vi "Main_21b.vi"() -> ()   [LabVIEW 2023]
uses:
  Cluster_Node.ctl
  ENUM Tile Marks.ctl
panel:
  out "left of set":i32
  out "Left of count":i32
  out "Array":T1[][](array[typedef])
  out "Start Point":T2
  out "Answer":i32
  in  "Puzzle":string="...................................................................................................................................\n.....#..#..#.#..#..#..#................##.#.......#....................#......#.##...........#.....##...................#........#.\n.....#.#.............#.............#.....#.........#..................................#......#....#...##...#.#........#......###...\n.......#...#................#.......#....#.....#...#.......................#......#...#.##...#.....#.........#.......#.#...........\n.##.............#...................#...#......#........#.........................#...#........#....#....#.........#..........#....\n.....#..##....#..#...#......##......#.................................................#.#.....#......#......#.#.##.................\n..............#......#......#................#.................#.................#................#..#...#........##.............#.\n..........##..........##.......#.#.....#..........#...#.........#.....................#....#....................#..#.....##..#..##.\n.#.#..#..#.#....#....#.....#...#.#.................................................#......................#..##..#.........#...#...\n.....................#.........#.......###..#......................#...........####........##.......#.#.#......#.#....##.....#...#.\n.#.#...#....#.........##...#...........#..##.......#.......#.......#................#.....#...#...#.#.....#..............##......#.\n................#...#..#.........#.##............................................#......##.....##.......#...#........#..#..#.......\n..#..#..####...###.#..........#........#.......#.............#.....#....#............#..#........##......##.......#.....#....#.....\n.......#..........#.......................#.............##..........#..#..........#.....#.............##.........#..............#..\n..................#.............##...........................#.#......##.......................##.....#.#.....#................#...\n.......#...................##........#...............................#..............#..#..#.#..#..........#........#...........#...\n...#..........#..#...#.#.#............................#......................#.......#......##...#...............#...#..#..........\n...#.#..........#.#.....#........#.....#...#.......................#.....#..#...............#.....#.#......#....##...#....#..###...\n...#.##........#..##...#..........#..#..................................#..#.#.#.........#...........#....#.....#...#.#.........#..\n.....#.......#........#..............#.##.............#..#........#....#.....#.............#....#.#.#........##........#...#..#....\n....#......##....##........#..#....##.................#......................#.#.#................#....#..###..#...#...............\n....#....#.#........#.......#........#...................#.....#.........#....#............##.........#..............#...........#.\n............#..#.##..................#..........##.........................#..#....#................#................#..#....#.....\n.##.##........#..###.......#....#......................##..#......#.....#...#..#...............##.#.....##........#................\n.......#..#........#.........#...................#..#.....##...............#.#.#...#..........#............#.....##.........#......\n...###.......#...............#...................#..#...##.........#.............##..#..........................#..#...#.....#.....\n..#..............##.........#..#...............................#........#......#.#....#..........#................##.#...#.........\n...#......#..#....#.........#..#..........##............#....#.........#....#..#......#.........#..#...........#...................\n.#...###.....................#.............#.......#......###..#...........#.........................#..#.......#.#..#.....#.......\n.###........#......##...#...........................##......#.........#.........#........#........#.....##..........#....#.........\n.......#........#..#......#..............#..........##...#...#...........................#...........#...#..#......#...........#...\n.#....#........#......#..##..................#....................#.................................#......#.....#..#.......#......\n...#........#.....#..##...#.#.............#...#.#.#.....#......#........#...........#....#...............#..#.....#.......#........\n....#....#...#.#....#................#..#......#........#.#........#..#.#..#..#.....#..#..................##...................#...\n.......##........#...#..............###.#....#....#..#....##...#....##.#............#..#.#...#............#...................#.#..\n..#......#.........#..#.................#...#.......#....#...#..............##...#..........#.#...........................#....#...\n..#......#..#...........................#...........#....#.............#.#.........#...#.........................##............#...\n.....#................#.........#.#.........#...........#.#............#..................#....#.........................#..#..#...\n......#...#....##...................#.................#..#........#..#..#.....................#.............#.......#..#......#....\n.............##.................#.......#.........#..#....#...#.......#...................#.........#.......##.#...................\n......#....#.................#..#....#..##..#............#..............#.............#.....#..#..#................#..#...#......#.\n..................#.........#.....................#......#....##..##...##..........#......#......#..#.............#.....#....#.....\n.......#...#..#....#..........#.......#.#.#...##.....##.#....#.##..................##........#...##..................#.............\n.............#...#..................#......##.........#.......##......#...#....##.....#...#..#...................#...####..........\n.............................#.......#....#........#..........#...#.......#.#............#..###........#...........#.#.............\n..........#...................#..#...............#.#..................#.....#...#..............................................##..\n.........................................#...#.#....#.......#........#..#......#.........#...............#.........................\n......#...#.......................#.....#................#.........#..#......#....................####.#..#.....................##.\n.......#...................#.##....#......#..........#...............##...#...#...............#.......#.....#.................#....\n....#.#...##............#.......#..........#..................#..........#.........#........#.........##...#.......................\n...#......#.........#........#....#.....#.........#....##....#..................#.......#.#.........#.#..................##....#...\n.....#................#.#...........#.............#..#.......#..........#..#...#.#.....###......##.....#.#.#.#.................#...\n.....................#..##.##...#...............#..#....#....#....#..####...#..................................#.........##..#.....\n.......##...............#......#.....#..........#..#..#.#.............#.....#......#.#.......#..................#............#..##.\n...#............#...#.........##............#...#...#......#.......#.....#...##...##...#...#................................#......\n...#.#.............................................##..............##..................#...........#...#..........#...........##...\n...#.#....................#......#....#.....##..........#.........#......#.#.......##.#.#....#.#....#.....#....##..................\n.............#...#.#..#......#........#.#...##.#...............#....#.........................#....#.......#.....##...#.........#..\n..................##..#..###......................#.......#.##.....#....#..#.....#....#..............#.....#.#..#....#.............\n.............#......#.###..###........#.#.#......#.#....#..#.......#..#............#.........#.#..#...............#.............##.\n.............#...#.............#.#.#..##..####..#......#.##.#...........##...##.............#......#.............#..#............#.\n..........#........#......#.#........#..............#......#..#.#.....#.................#...#...............#.#..........##........\n..............#.............##.....#............................#..........#..........#..#.....................#..#..#.............\n..........#...#.#.......##....#.......#..##......#...#.....#............#................#....#.......................#............\n....................#.....#..........#.......#.#........#...##..............#.....#.......#..##...#..#####.#.#.........##....#.....\n.................................................................S.................................................................\n........#.........##....#........#...........................##........#..............#........#.....#.#..............#....#.......\n......#............#.............#............#.##...........#..#.....#....#.....#......#.#.#.......#.#.#...#......................\n............................#.........#........###........#...#....#.........#................#..#.............#....#..............\n............#......##..##.##...##.............#.........#............#.###.....#..................##..................#..#.........\n..............#......#................#...............#.....##..#..........#.....#..#..........#...........#.......................\n.........................#...........#..#......#.............#..#....#.......#..#.....#...#.............................#........#.\n...........##.....##.................#..........#.#.#..............#.....#.........#............#.................#................\n.........................#......#.....#...#.##...........#......#....#....#......#..#.#..#..###..##.##.....#...................#...\n.....#...........#.....#.......#..##......##.#.#.#..........#..#..............#...#.#.#.....#............#.#....#..............#.#.\n...#...........#.........#..#.#.#.........#........#..#........................#..........#.............#....##.#...............#..\n...............#.....................................#..............................##...###.................#..#..........#.....#.\n........#..........#..#......###............#........................#..........#............................................#.....\n...............................#....................#..................................##.............#............................\n.........#............#..#..........#........#..#...##....#....#..#......#.....#.#...#......................##..................#..\n......##.#..........##.#..................................#.........#......##..#...............#........#.....#............#.......\n.........#..................#...........#.#.......................#..........#.......##.......#.....#...##...#........#...#.#......\n...#...................#.....#...........##............#..#...#..................#.#..........#........................#...........\n..#.........#.........#.........##...#.....#...........#.....................#....#............#..#.......#.........#.....#........\n..........#....#..........#.........#..........#..###........#.#..........##.................#......#...#..............#...........\n..#....##..........................#..........#........#.#..##..#.....#.#....#..#.....................#............#.#...........#.\n.....................................#..#.#..#...........#...#.#.......#........#...#.........#...#..#...............#.............\n.........#.#....##.................#.#.....#....#..#..#................#...##.......#...........#.....#.................##.........\n..#.........................#......#..............#.............#.......#.............#........#................#...###.#........#.\n.#..#............#..............#..#...........#................#.........#....#................#..#.............#.....#...#.....#.\n.....#.......................#............#...............#..........###.....##...........#..#...#.##.........#.......#............\n.#..#..........#.............................#......#.......##..........#.........#....#...#.....#..........#....#.................\n.........#.......................#.##.....#.....#.#....#.......##.....#....#......#.......#.#.....................#.##..#..#....#..\n.#......#.....#.....#.....................##.........#....#...##..#..................##...#.#.#..#........#..#.........#.#....#.##.\n.#...............................#.#.#..#..##.....#........#...#.....#..#...#......#.#....#...##..................#................\n...........#......#...............#.....#.....#..##.........##........#.....#.........#...#..#............#.#.#...........#........\n..#............#..##..#..#..........#...#.......#.........#.......#.....#............................................#....#...#.#..\n....#...........#....................#............................#.#...#...............#.#..#.....................................\n.....##......#.##...#............................#........#...#...........#.........#......##...........#.#..#...............#.....\n......#..............##.#.###...........#.....#.#.##....#..#..........#...#..#..............................#.....#..............#.\n..##.....................##...............#...#......#........#..................#............................#.###..#...#....#..#.\n........#.#............#....................##.....#..........#...................#...#..#...........#........#.........#....##....\n.....#....#..#...............#............#.....#.......#...#........#............#..##.............#.......................#......\n..#.........#.............#...........................#.......#.#.................#..###.........................#.#.#.#.....#.....\n....#...#.................#................#........#..........#..........#.......#..........................#.#......#.......#....\n......#..##........#....#........................#.........#.........#................#......................#........#.....#....#.\n............#......#.........................................##......#.#..#.........#.............##..........#............#.......\n......#.#....#....#......#......##................#........#......#....#.....#....#.#..............#.......#.#...#......#......#...\n.....#............##.....#........#.#..#.........#.#................#...#.........#...........#.....#..#............#.....#..#.#...\n.......##..#........#..#..#.......................#............................................................#...#.#.....#.......\n....#...............#.......#............#.................#..............#..#...........#.......#............#................#...\n.......#.........##.......................#.......#....#......###...#....#..#................##...#.................#.#............\n...#.#.......#........#..#...........................#......#.....#.........##..........#..........##..............#....#........#.\n..#.#...........##..........#...#.........#..........#.#............##..................................#...........##.............\n.#..............#.........##.#.##..#...#....#.............#..............#............#..................#.#........#..............\n..#..#.....#....#.........#..#.#......#..#...#.............#..........#.................#...##.....#..........#...............#....\n......#.........#..#.#.....#................#......................#...##...........#..#................#.............#....##....#.\n...................#.....#.........##.....##...........................#....................#......#..................#..#.#.......\n..#............#...........##.#................................#............................#.........................#...#....#...\n.....#............#..............#......#..#....................#............................#....#....................#....#..#...\n..........#..#.#.#..............#.................................................................#...............##...........#...\n........##.................#..........#.....##....#.........#..#...#.##.....................#..#.........................#.......#.\n....##.........#.....#.....................#..#.##...........#..#.........................#..........#.....#........#....##......#.\n..............#.......#........#.......#..##...................#...#....................#...........#....#.........................\n...............#.............##......#.##.#............#...................#....#..............#...#..#.#.....#...............#....\n.....#..............#...#.......##..........#......#...#..................#..................#........#....#.........#.............\n.#.......#.#......#........................#..#......#......................#......##....##..#..........#...................#......\n..........#...........#..#..###........#.#......#.....................................#####.......##........#.....#.......#........\n..##................#............#..........#...##....#........................#....#........#....#.##......#.........##....#......\n.........#....#.....#....#.#...##..........#.........#.#.................##..............#..#......#.......#...#..............#.#..\n..................................................................................................................................."
  in  "Example":string="...........\n.....###.#.\n.###.##..#.\n..#.#...#..\n....#.#....\n.##..S####.\n.##..#...#.\n.......##..\n.##.#.####.\n.##..##.##.\n..........."
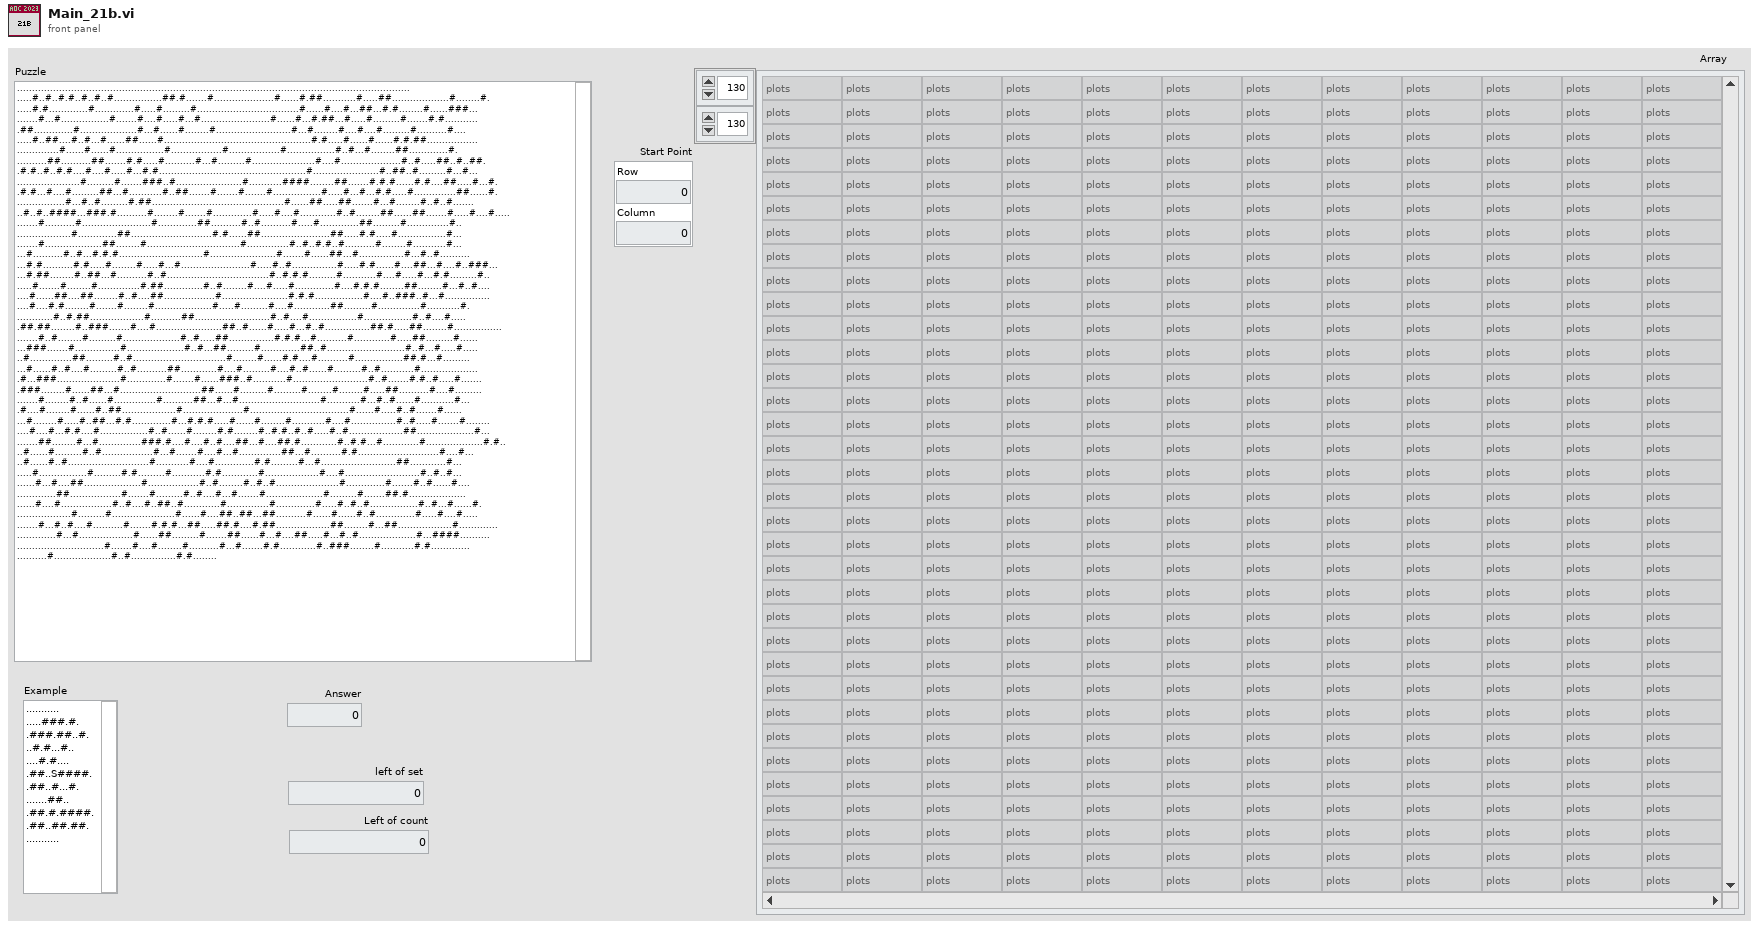
[diagram p1: front panel]
types:
  T1 = typedef "ENUM Tile Marks.ctl" = enum16{"plots", "rocks", "Start", "Marked Tiles"}
  T2 = typedef "Cluster_Node.ctl" = cluster{"Row":i32, "Column":i32}
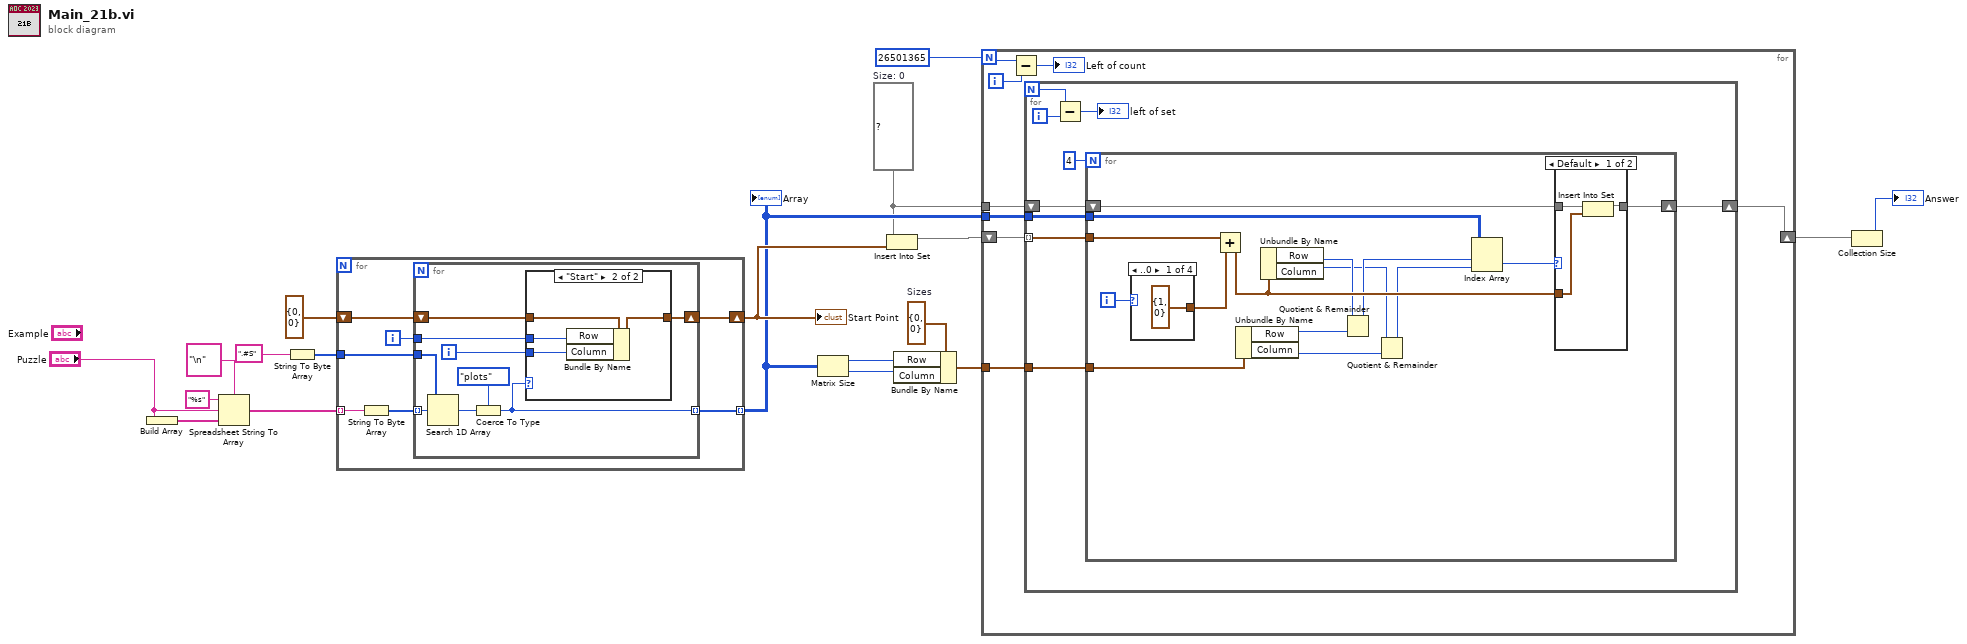
[diagram p0: block diagram]
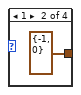
[diagram p2: hidden frame]
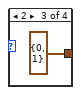
[diagram p3: hidden frame]
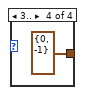
[diagram p4: hidden frame]
diagram:
  w8 = T2 {"Row"=0, "Column"=0}  # Sizes
  w7 = set{T2} {}  # Size: 0
  n1 = Build Array("Puzzle") -> (w19:string[])
  n2 = Spreadsheet String To Array(delimiter (Tab)="\n", format string="%s", spreadsheet string="Puzzle", array type (2D Dbl)=w19) -> (array=w16:string[])
  n3 = String To Byte Array(string=".#S" ("format string")) -> (unsigned byte array=w14:u8[])
  n4 = for {
    tunnel: w16 -> [w26] mode=indexing
    tunnel: w14 -> [w25]
    tunnel: [w23] -> w9 mode=indexing
    shift-right: [w20] -> w10
    shift-left: T2 {"Row"=0, "Column"=0} ("Point") -> [w22]
    i -> [w21]
    n5 = String To Byte Array(string=w26) -> (unsigned byte array=w24:u8[])
    n6 = for {
      tunnel: w25 -> [w35]
      tunnel: w24 -> [w34] mode=indexing
      tunnel: [w31] -> w23 mode=indexing
      shift-right: [w27] -> w20
      shift-left: w22 -> [w30]
      tunnel: w21 -> [w29]
      i -> [w28]
      n7 = Search 1D Array(1D array=w35, element=w34) -> (index of element=w33:i32)  [unwired: 1 in]
      n8 = Coerce To Type(0:w33, 1:ENUM_Tile_Marks."plots") -> (2:w31:T1)
      n9 = case shown="\"Start\"" w31 {
        tunnel: w30 -> [w36 w40]
        tunnel: w29 -> [_ w38]
        tunnel: w28 -> [_ w37]
        tunnel: [w36 w39] -> w27
        frame Default {
        }
        frame "Start" {
          n10 = Bundle By Name(cluster=w40, "Row"=w38, "Column"=w37) -> (w39:T2)
        }
      }
    }
  }
  "Start Point" <- w10
  "Array" <- w9
  n11 = Matrix Size(0:w9) -> (1:w1:i32, 2:w2:i32)
  n12 = Insert Into Set(10:w10, 11:w7) -> (3:w11:set{T2})  [unwired: 1 out]
  n13 = Bundle By Name(cluster=w8, "Row"=w1, "Column"=w2) -> (w3:T2)
  n14 = for {
    N: 26501365 -> [w44]
    tunnel: w9 -> [w47]
    shift-right: [w45] -> w6
    shift-left: w11 -> [w48]
    tunnel: w7 -> [w46]
    tunnel: w3 -> [w41]
    i -> [w43]
    n15 = Subtract(x=w44, y=w43) -> (x-y=→"Left of count":i32)
    n16 = for {
      N -> [w51]
      tunnel: w48 -> [w56] mode=indexing
      tunnel: w47 -> [w55]
      shift-right: [w53] -> w45
      shift-left: w46 -> [w54]
      tunnel: w41 -> [w49]
      i -> [w52]
      n17 = Subtract(x=w51, y=w52) -> (x-y=→"left of set":i32)
      n18 = for {
        N: 4 -> [_]
        tunnel: w56 -> [w71]
        tunnel: w55 -> [w69]
        shift-right: [w66] -> w53
        shift-left: w54 -> [w67]
        tunnel: w49 -> [w64]
        i -> [w72]
        n19 = case shown="..0" w72 {
          tunnel: [T2 {"Row"=1, "Column"=0} ("Start Point 2") T2 {"Row"=-1, "Column"=0} ("Start Point 2") T2 {"Row"=0, "Column"=1} ("Start Point 2") T2 {"Row"=0, "Column"=-1} ("Start Point 2")] -> w70
          frame ..0 {
          }
          frame 1 {
          }
          frame 2 {
          }
          frame 3.. {
          }
        }
        n20 = Add(x=w71, y=w70) -> (x+y=w68:T2)
        n21 = Unbundle By Name(w64) -> ("Row"=w63:i32, "Column"=w62:i32)
        n22 = Unbundle By Name(w68) -> ("Row"=w61:i32, "Column"=w59:i32)
        n23 = Quotient & Remainder(x=w61, y=w63) -> (x-y*floor(x/y)=w60:i32)  [unwired: 1 out]
        n24 = Quotient & Remainder(x=w59, y=w62) -> (x-y*floor(x/y)=w58:i32)  [unwired: 1 out]
        n25 = Index Array(array=w69, index (row)=w60, index (col)=w58) -> (element=w65:T1)
        n26 = case shown="Default" w65 {
          tunnel: w67 -> [w79 w80]
          tunnel: [w78 w80] -> w66
          tunnel: w68 -> [w77 _]
          frame Default {
            n27 = Insert Into Set(10:w77, 11:w79) -> (3:w78:set{T2})  [unwired: 1 out]
          }
          frame "rocks" {
          }
        }
      }
    }
  }
  n28 = Collection Size(1:w6) -> (0:→"Answer":i32)
